vi "PH_Timing.Action link Sequencer.vi"(0 "i ref in":refnum<vi>, 5 "error in (no error)":errorcluster) -> (14 "i ref out":refnum<vi>, 19 "error out":errorcluster)   [LabVIEW 2014, in "PH_Timing.lvlib"]
uses:
  PH_Timing.lvlib
  PH_Common/PH_Common.lvlib
  CSDigitalIO/BNC555/BNC555.lvlib
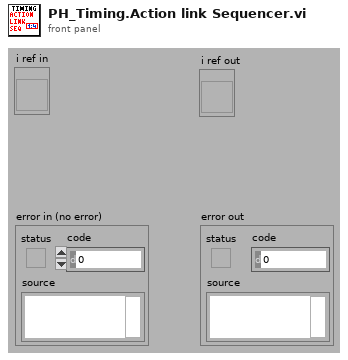
[diagram p1: front panel]
types:
  T1 = typedef "PH_Timing.lvlib/PH_Timing.i attribute.ctl" = cluster{"Sequencer":cluster{"linked?":bool, "Proc State":string, "Ref State":refnum<vi>}, "Gate Generator":cluster{"GD":cluster{"Device Status":T2, "linked?":bool}, "Settings":T3, "GUI Ref":refnum<vi>}, "Interlock Bypass":cluster{"Instancename":string, "Switch linked?":bool, "Device Status":T2, "Ref Status":refnum<vi>}, "Roughtuner":cluster{"Settings":T4, "GUI Ref":refnum<vi>, "GD":cluster{"Device Status":T2, "linked?":bool}}, "0,5Hz Gater":cluster{"Settings":T5, "GUI Ref":refnum<vi>, "GD":cluster{"Device Status":T2, "linked?":bool}}, "Slow Trigger":cluster{"Settings":T6, "GUI Ref":refnum<vi>, "Service ID Delay":i32, "Service ID Ext Trig":i32, "Wanted Settings":T6}, "Timing Mode":cluster{"Mode":T7, "GUI Ref":refnum<vi>, "Service ID T2":i32, "Service ID Mode":i32, "Wanted Mode":T7}, "ns Generator":cluster{"Settings":T8, "ns Generator Settings":refnum<vi>, "GD":cluster{"Device Status":T2, "linked?":bool}}, "Phase FEs":cluster{"Settings":T11, "GUI Ref":refnum<vi>, "Service ID Phase":i32, "Wanted Settings":T11}, "GD GUI Refs":refnum<vi>[], "Heads":T12[], "GUI Ref Delete":refnum<vi>}
  T2 = typedef "PH_StatusHandler.lvlib/PH_StatusHandler.Status.ctl" = i16
  T3 = typedef "PH_Timing.lvlib/PH_Timing.GateGen.ctl" = cluster{"Instance":string, "Channel Gate":i32, "Channel T2":i32, "Width Gate":dbl, "Width T2":dbl, "Delay Gate":dbl, "Delay T2":dbl, "Gate activ":bool, "T2 activ":bool, "System Mode":enum16{"Normal", "Single", "Burst", "Duty Cycle"}}
  T4 = typedef "PH_Timing.lvlib/PH_Timing.Roughtuner.ctl" = cluster{"Instance":string, "Phase PHELIX / UNILAC":cluster{"Channel":u16, "relative to":u16, "Delay [ms]":dbl}, "Pulse Length":cluster{"Channel":u16, "relative to":u16, "Delay [ms]":dbl}, "Trigger":cluster{"externally?":bool, "Rate [Hz]":dbl}}
  T5 = typedef "PH_Timing.lvlib/PH_Timing.0.5HzGater.ctl" = cluster{"Instance":string, "Channel ns FE Delay":i32, "Channel 0.5Hz":i32, "Width ns FE Delay":dbl, "Width 0.5Hz":dbl, "Delay ns FE Delay":dbl, "Delay 0.5Hz":dbl, "ns FE Delay active":bool, "0.5Hz activ":bool, "ns FE Delay inverted":bool, "0.5Hz inverted":bool}
  T6 = typedef "PH_Timing.lvlib/PH_Timing.Slow Trigger Settings.ctl" = cluster{"Delay":dbl, "externally triggered?":bool}
  T7 = typedef "PH_Timing.lvlib/PH_Timing.Timing Mode.ctl" = cluster{"T2":i16, "Modeselector":enum32{"10 Hz", "0.5 Hz", "Shot"}}
  T8 = typedef "PH_Timing.lvlib/PH_Timing.ns Generator.ctl" = cluster{"Instance":string, "Phase fs / ns FE":cluster{"Channel":T9, "Settings":T10}}
  T9 = typedef "Stanford Research DG645 - Driver.lvlib/Channel.ctl" = i32
  T10 = typedef "PH_SRDG645.lvlib/PH_SRDG645.Channel Settings.ctl" = cluster{"Delay [s]":dbl, "relative to":i32}
  T11 = typedef "PH_Timing.lvlib/PH_Timing.Phase FEs.ctl" = cluster{"Phase":dbl}
  T12 = typedef "PH_Timing.lvlib/PH_Timing.PU Data.ctl" = cluster{"linked?":bool, "Data":T13, "GD":cluster{"Device Status":T2, "linked?":bool}, "GUI Ref":refnum<vi>, "PU":T14}
  T13 = typedef "PH_Timing.lvlib/PH_Timing.PU Info.ctl" = cluster{"Act CH?":bool, "GD":string, "CH":i32, "Delay":dbl, "active":bool, "in Use?":bool}
  T14 = typedef "PH_PP_Common.lvlib/PH_PP_Common.PUs.ctl" = enum16{"no Info", "PA-19mm-1", "PA-19mm-2", "PA-45mm-PILC", "PA-45mm-MAIN", "MA-PU-1", "MA-PU-2", "MA-PU-3", "MA-PU-4", "MA-PU-5", "MA-PU-6", "MA-FR", "MA-PILC", "PA-45mm-DP"}
  T15 = cluster{"GD":cluster{"Device Status":T2, "linked?":bool}, "Settings":T3, "GUI Ref":refnum<vi>}
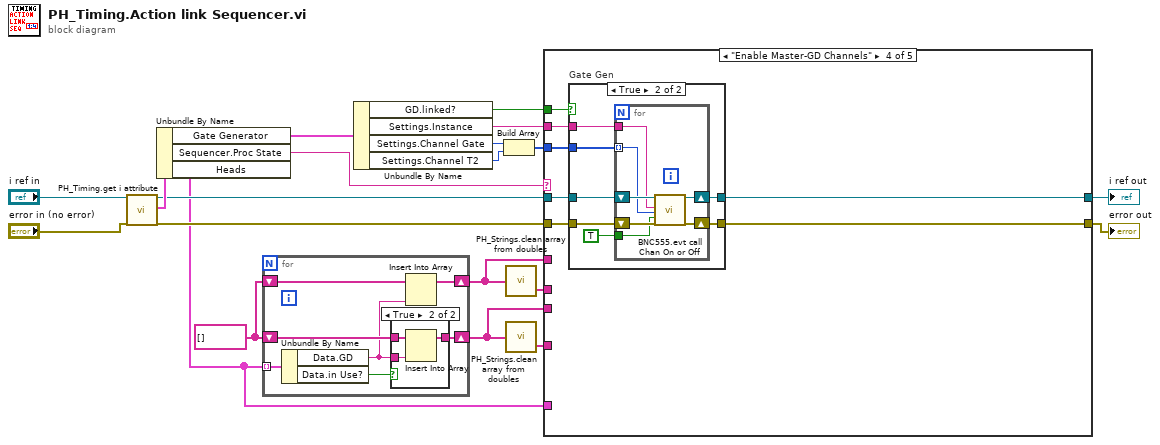
[diagram p0: block diagram]
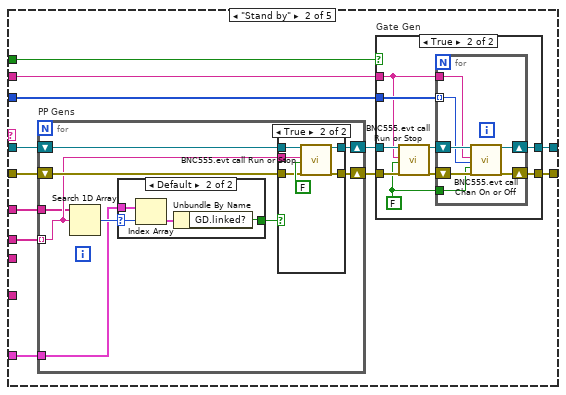
[diagram p4: hidden frame]
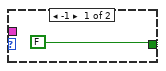
[diagram p6: hidden frame]
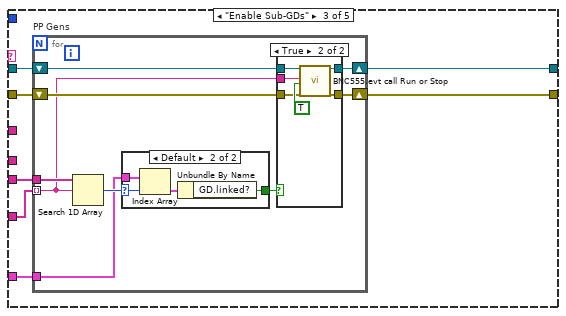
[diagram p8: hidden frame]
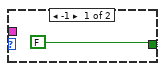
[diagram p9: hidden frame]
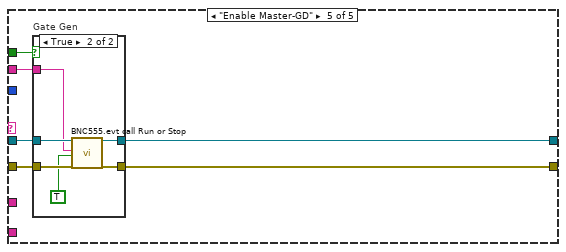
[diagram p12: hidden frame]
diagram:
  w7 = string[] []
  n1 = call "PH_Timing.get i attribute.vi"("i ref in"="i ref in", "error in (no error)"="error in (no error)") -> ("i ref out"=w17:refnum<vi>, "i attribute"=w20:T1, "error out"=w15:errorcluster)  [unwired: 15 in]
  n2 = Unbundle By Name(w20) -> ("Gate Generator"=w12:T15, "Sequencer.Proc State"=w13:string, "Heads"=w1:T12[])
  n3 = for {
    tunnel: w1 -> [w27] mode=indexing
    shift-right: [w26] -> w3
    shift-left: w7 -> [w24]
    shift-right: [w25] -> w4
    shift-left: w7 -> [w23]
    n4 = Unbundle By Name(w27) -> ("Data.GD"=w22:string, "Data.in Use?"=w21:bool)
    n5 = case shown="True" w21 {
      tunnel: [w28 w31] -> w26
      tunnel: w22 -> [_ w30]
      tunnel: w24 -> [w28 w29]
      frame False {
      }
      frame True {
        n6 = Insert Into Array(array=w29, new element=w30) -> (w31:string[])  [unwired: 1 in]
      }
    }
    n7 = Insert Into Array(array=w23, new element=w22) -> (w25:string[])  [unwired: 1 in]
  }
  n8 = Unbundle By Name(w12) -> ("GD.linked?"=w2:bool, "Settings.Instance"=w8:string, "Settings.Channel Gate"=w11:i32, "Settings.Channel T2"=w10:i32)
  n9 = Build Array(w11, w10) -> (w9:i32[])
  n10 = call "PH_Strings.clean array from doubles.vi"("Array Input"=w4) -> ("Cleaned Array Output"=w6:string[])  [unwired: 1 out]
  n11 = call "PH_Strings.clean array from doubles.vi"("Array Input"=w3) -> ("Cleaned Array Output"=w5:string[])  [unwired: 1 out]
  n12 = case "Seq States" shown="\"Enable Master-GD Channels\"" w13 {
    tunnel: w17 -> [w32 w39 w91 w116 w139]
    tunnel: [w32 w45 w89 w120 w142] -> w16
    tunnel: w15 -> [w33 w37 w92 w117 w140]
    tunnel: [w33 w41 w90 w121 w143] -> w14
    tunnel: w2 -> [_ w44 _ w119 w141]
    tunnel: w9 -> [_ w43 _ w118 _]
    tunnel: w8 -> [_ w42 _ w115 w138]
    tunnel: w6 -> [_ w40 _ _ _]
    tunnel: w5 -> [_ _ w88 _ _]
    tunnel: w4 -> [_ w35 _ _ _]
    tunnel: w1 -> [_ w34 w86 _ _]
    tunnel: w3 -> [_ _ w87 _ _]
    frame Default {
    }
    frame "Stand by" {
      n13 = for "PP Gens" {
        tunnel: w40 -> [w49] mode=indexing
        shift-right: [w52] -> w38
        shift-left: w39 -> [w53]
        shift-right: [w50] -> w36
        shift-left: w37 -> [w51]
        tunnel: w35 -> [w48]
        tunnel: w34 -> [w46]
        n14 = Search 1D Array(1D array=w48, element=w49) -> (index of element=w47:i32)  [unwired: 1 in]
        n15 = case shown="Default" w47 {
          selector: w47 -> [_ w65]
          tunnel: w46 -> [_ w67]
          tunnel: [FALSE ("linked?") w64] -> w54
          frame -1 {
          }
          frame Default {
            n16 = Index Array(array=w67, index=w65) -> (element=w66:T12)
            n17 = Unbundle By Name(w66) -> ("GD.linked?"=w64:bool)
          }
        }
        n18 = case shown="True" w54 {
          tunnel: w53 -> [w56 w61]
          tunnel: [w56 w60] -> w52
          tunnel: w51 -> [w55 w59]
          tunnel: [w55 w57] -> w50
          tunnel: w49 -> [_ w58]
          frame False {
          }
          frame True {
            n19 = call "BNC555.evt call Run or Stop.vi"("i ref in"=w61, "Generator Instance"=w58, "Start\\Stop"=FALSE, "error in (no error)"=w59) -> ("i ref out"=w60:refnum<vi>, "error out"=w57:errorcluster)  [unwired: 14 in]
          }
        }
      }
      n20 = case "Gate Gen" shown="True" w44 {
        tunnel: w36 -> [w68 w76]
        tunnel: [w68 w71] -> w41
        tunnel: w38 -> [w69 w74]
        tunnel: [w69 w78] -> w45
        tunnel: w43 -> [_ w77]
        tunnel: w42 -> [_ w72]
        frame False {
        }
        frame True {
          w73 = FALSE
          n21 = call "BNC555.evt call Run or Stop.vi"("i ref in"=w74, "Generator Instance"=w72, "Start\\Stop"=w73, "error in (no error)"=w76) -> ("i ref out"=w75:refnum<vi>, "error out"=w70:errorcluster)  [unwired: 14 in]
          n22 = for {
            tunnel: w73 -> [w81]
            shift-right: [w83] -> w78
            shift-left: w75 -> [w84]
            shift-right: [w79] -> w71
            shift-left: w70 -> [w85]
            tunnel: w72 -> [w82]
            tunnel: w77 -> [w80] mode=indexing
            n23 = call "BNC555.evt call Chan On or Off.vi"("i ref in"=w84, "Generator Instance"=w82, "Channel"=w80, "State"=w81, "error in (no error)"=w85) -> ("i ref out"=w83:refnum<vi>, "error out"=w79:errorcluster)  [unwired: 13 in]
          }
        }
      }
    }
    frame "Enable Sub-GDs" {
      n24 = for "PP Gens" {
        tunnel: w88 -> [w95] mode=indexing
        shift-right: [w100] -> w89
        shift-left: w91 -> [w101]
        shift-right: [w98] -> w90
        shift-left: w92 -> [w99]
        tunnel: w87 -> [w96]
        tunnel: w86 -> [w94]
        n25 = Search 1D Array(1D array=w96, element=w95) -> (index of element=w97:i32)  [unwired: 1 in]
        n26 = case shown="Default" w97 {
          selector: w97 -> [_ w104]
          tunnel: w94 -> [_ w106]
          tunnel: [FALSE ("linked?") w103] -> w93
          frame -1 {
          }
          frame Default {
            n27 = Index Array(array=w106, index=w104) -> (element=w105:T12)
            n28 = Unbundle By Name(w105) -> ("GD.linked?"=w103:bool)
          }
        }
        n29 = case shown="True" w93 {
          tunnel: w101 -> [w108 w113]
          tunnel: [w108 w112] -> w100
          tunnel: w99 -> [w107 w111]
          tunnel: [w107 w109] -> w98
          tunnel: w95 -> [_ w110]
          frame False {
          }
          frame True {
            n30 = call "BNC555.evt call Run or Stop.vi"("i ref in"=w113, "Generator Instance"=w110, "Start\\Stop"=TRUE, "error in (no error)"=w111) -> ("i ref out"=w112:refnum<vi>, "error out"=w109:errorcluster)  [unwired: 14 in]
          }
        }
      }
    }
    frame "Enable Master-GD Channels" {
      n31 = case "Gate Gen" shown="True" w119 {
        tunnel: w117 -> [w122 w125]
        tunnel: [w122 w124] -> w121
        tunnel: w116 -> [w123 w126]
        tunnel: [w123 w130] -> w120
        tunnel: w118 -> [_ w129]
        tunnel: w115 -> [_ w127]
        frame False {
        }
        frame True {
          n32 = for {
            tunnel: TRUE -> [w133]
            shift-right: [w135] -> w130
            shift-left: w126 -> [w136]
            shift-right: [w131] -> w124
            shift-left: w125 -> [w137]
            tunnel: w127 -> [w134]
            tunnel: w129 -> [w132] mode=indexing
            n33 = call "BNC555.evt call Chan On or Off.vi"("i ref in"=w136, "Generator Instance"=w134, "Channel"=w132, "State"=w133, "error in (no error)"=w137) -> ("i ref out"=w135:refnum<vi>, "error out"=w131:errorcluster)  [unwired: 13 in]
          }
        }
      }
    }
    frame "Enable Master-GD" {
      n34 = case "Gate Gen" shown="True" w141 {
        tunnel: w140 -> [w144 w151]
        tunnel: [w144 w146] -> w143
        tunnel: w139 -> [w145 w150]
        tunnel: [w145 w149] -> w142
        tunnel: w138 -> [_ w147]
        frame False {
        }
        frame True {
          n35 = call "BNC555.evt call Run or Stop.vi"("i ref in"=w150, "Generator Instance"=w147, "Start\\Stop"=TRUE, "error in (no error)"=w151) -> ("i ref out"=w149:refnum<vi>, "error out"=w146:errorcluster)  [unwired: 14 in]
        }
      }
    }
  }
  "error out" <- w14
  "i ref out" <- w16
